vi "readfeedback.vi"(0 "object in":refnum<class "MBinteractive.lvclass">, 5 "error in (no error)":errorcluster) -> (14 "object out":refnum<class "MBinteractive.lvclass">, 15 "feedback":u16, 19 "error out":errorcluster)   [LabVIEW 2016, in "MBinteractive.lvclass"]
uses:
  MBinteractive.lvclass
  MBinteractive.lvclass/MBinteractive.ctl
  <vilib>/NI/Modbus Library/API/Modbus API.lvclass
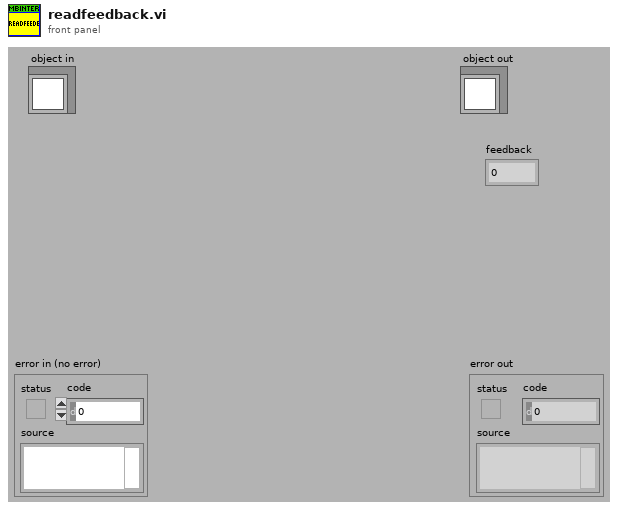
[diagram p1: front panel]
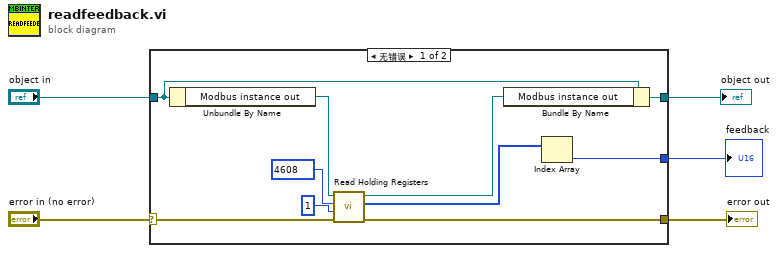
[diagram p0: block diagram]
diagram:
  n1 = case shown="无错误" "error in (no error)" {
    selector: "error in (no error)" -> [w11 w17]
    tunnel: [w10 w17] -> w4
    tunnel: [w9 w16] -> w2
    tunnel: "object in" -> [w15 w16]
    tunnel: [w6 _] -> w1
    frame No Error {
      n2 = Unbundle By Name(w15) -> ("Modbus instance out"=w12:refnum<class "Modbus API.lvclass">)
      n3 = call-dynamic "Read Holding Registers.vi"("error in"=w11, "number of inputs"=u16 1 ("number of holding registers"), "starting address"=u16 4608, "Modbus instance in"=w12) -> ("error out"=w10:errorcluster, "register values"=w7:u16[], "Modbus instance out"=w8:refnum<class "Modbus API.lvclass">)  [unwired: 5 in]
      n4 = Bundle By Name(cluster=w15, "Modbus instance out"=w8) -> (w9:refnum<class "MBinteractive.lvclass">)
      n5 = Index Array(array=w7) -> (element=w6:u16)  [unwired: 1 in]
    }
    frame Error {
    }
  }
  "error out" <- w4
  "object out" <- w2
  "feedback" <- w1
